vi "TDMS delete channel.vi"(7 "Delay":u32=10 format="%.0fms", 8 "error in (no error)":errorcluster, 9 "Channels":string[](array[string]), 10 "group name":string="Untitled", 11 "file path":path) -> (0 "error out":errorcluster, 1 "Deleted channels":string[](array[string]), 3 "file path out":path)   [LabVIEW 2018]
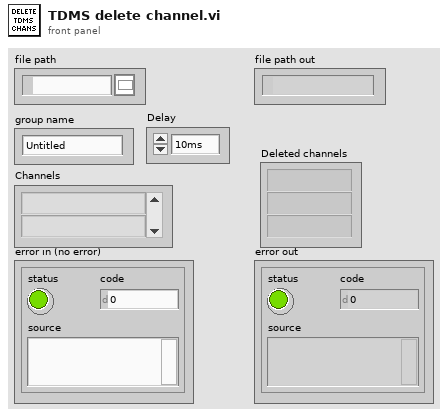
[diagram p1: front panel]
types:
  T1 = enum16{"open", "open or create", "create or replace", "create", "open (read-only)"}
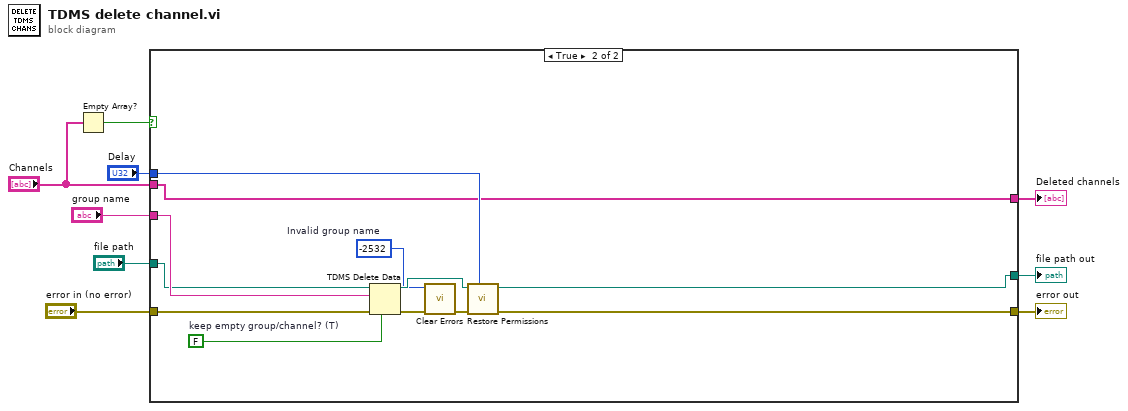
[diagram p0: block diagram]
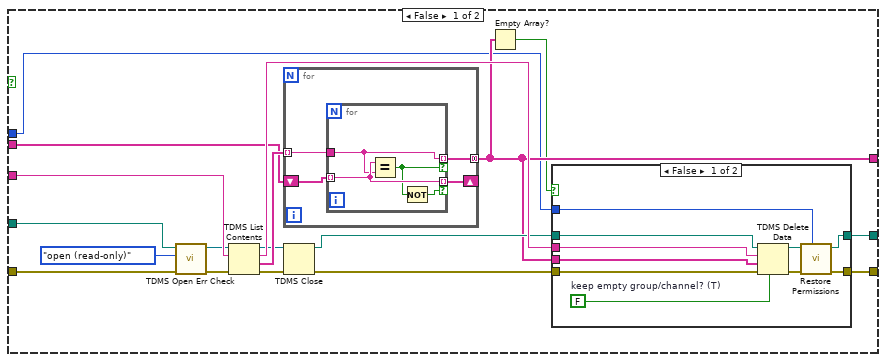
[diagram p2: hidden frame]
diagram:
  n1 = Empty Array?(array="Channels") -> (empty?=w1:bool)
  n2 = case shown="True" w1 {
    tunnel: "group name" -> [w27 w59]
    tunnel: [w20 w58] -> w8
    tunnel: [w19 w57] -> w7
    tunnel: [w18 w51] -> w6
    tunnel: "Delay" -> [w16 w56]
    tunnel: "file path" -> [w14 w50]
    tunnel: "error in (no error)" -> [w13 w55]
    tunnel: "Channels" -> [w10 w51]
    frame False {
      n3 = call "TDMS Open Err Check.vi"("Error In"=w13, "operation (0:open)"=T1."open (read-only)", "File Path Control"=w14) -> ("Error Out"=w12:errorcluster, "tdms file out"=w11:refnum<k34>)  [unwired: 6 in, 1 out]
      n4 = TDMS List Contents(4:w12, 6:w27, 7:w11) -> (0:w24:errorcluster, 1:w26:string[], 2:w25:string, 3:w23:refnum<k34>)
      n5 = for {
        tunnel: w26 -> [w42] mode=indexing
        shift-right: [w41] -> _
        shift-left: w10 -> [w43]
        tunnel: [w40] -> w18 mode=concatenating
        n6 = for {
          tunnel: w43 -> [w47] mode=indexing
          tunnel: w42 -> [w45]
          tunnel: [w47] -> w41 mode=indexing if=w46
          tunnel: [w45] -> w40 mode=indexing if=w44
          n7 = Equal?(x=w47, y=w45) -> (x = y?=w44:bool)
          n8 = Not(x=w44) -> (.not. x?=w46:bool)
        }
      }
      n9 = TDMS Close(8:w24, 11:w23) -> (0:w21:errorcluster, 3:w22:path)
      n10 = Empty Array?(array=w18) -> (empty?=w17:bool)
      n11 = case shown="False" w17 {
        tunnel: w18 -> [w37 _]
        tunnel: w25 -> [w36 _]
        tunnel: w22 -> [w35 w38]
        tunnel: w21 -> [w34 w39]
        tunnel: [w31 w38] -> w20
        tunnel: [w29 w39] -> w19
        tunnel: w16 -> [w28 _]
        frame False {
          w33 = FALSE  # keep empty group/channel? (T)
          n12 = TDMS Delete Data(6:w33, 8:w34, 9:w37, 10:w36, 11:w35) -> (0:w30:errorcluster, 3:w32:path)  [unwired: 2 in]
          n13 = call "Restore Permissions.vi"("Delay"=w28, "Error In"=w30, "File Path"=w32) -> ("Error Out"=w29:errorcluster, "Duplicate File Path"=w31:path)  [unwired: 5 in, 2 out]
        }
        frame True {
        }
      }
    }
    frame True {
      w48 = -2532  # Invalid group name
      w54 = FALSE  # keep empty group/channel? (T)
      n14 = TDMS Delete Data(6:w54, 8:w55, 10:w59, 11:w50) -> (0:w52:errorcluster, 3:w53:path)  [unwired: 3 in]
      n15 = call <vilib>:"Clear Errors.vi"("error in (no error)"=w52, "specific error code to clear (0: all)"=w48) -> ("error out"=w49:errorcluster)  [unwired: 4 in, 1 out]
      n16 = call "Restore Permissions.vi"("Delay"=w56, "Error In"=w49, "File Path"=w53) -> ("Error Out"=w57:errorcluster, "Duplicate File Path"=w58:path)  [unwired: 5 in, 2 out]
    }
  }
  "file path out" <- w8
  "error out" <- w7
  "Deleted channels" <- w6
